vi "Write Suggestion Listbox.vi"(8 "error in (no error)":errorcluster, 10 "Suggestions ctrl":refnum<vi>, 11 "Static Listbox IO in":refnum<class "Static Listbox IO.lvclass">) -> (0 "error out":errorcluster, 3 "Static Listbox IO out":refnum<class "Static Listbox IO.lvclass">)   [LabVIEW 2016, in "Static Listbox IO.lvclass"]
uses:
  Static Listbox IO.lvclass
  Static Listbox IO.lvclass/Static Listbox IO.ctl
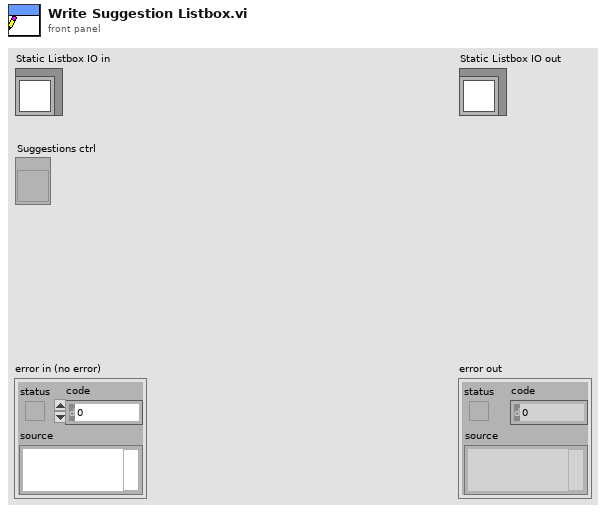
[diagram p1: front panel]
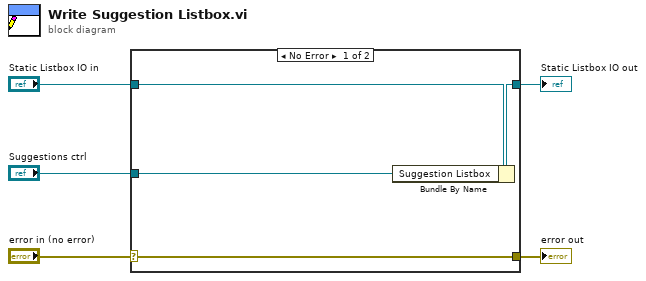
[diagram p0: block diagram]
diagram:
  n1 = case shown="No Error" "error in (no error)" {
    selector: "error in (no error)" -> [w9 w10]
    tunnel: [w9 w10] -> w4
    tunnel: [w7 w11] -> w2
    tunnel: "Static Listbox IO in" -> [w8 w11]
    tunnel: "Suggestions ctrl" -> [w6 _]
    frame No Error {
      n2 = Bundle By Name(cluster=w8, "Suggestion Listbox"=w6) -> (w7:refnum<class "Static Listbox IO.lvclass">)
    }
    frame Error {
    }
  }
  "error out" <- w4
  "Static Listbox IO out" <- w2
